vi "引用測試2.vi"() -> ()   [LabVIEW 2015]
uses:
  <vilib>/vision/Measure.llb/Edge Options.ctl
  <vilib>/vision/Measure.llb/Edge Polarity.ctl
  <vilib>/userdefined/High Color/IMAQdx.ctl
  <vilib>/vision/driver/NI_Vision_Acquisition_Software.lvlib
  <vilib>/vision/NI_Vision_Development_Module.lvlib
panel:
  in  "Boolean":bool
  out "Line Data":T1
  in  "取像":bool
  in  "Edge Options":T2={"Edge Polarity"=0, "Kernel Size"=3, "Width"=3, "Minimum Edge Strength"=10.0, "Interpolation Type"=enum."Bilinear Fixed", "Data Processing Method"=enum."Average"} {"Edge Polarity" items=["All Edges", "Rising Edges", "Falling Edges"]; "Minimum Edge Strength" format="%.2f"; "Width" step=2; "Kernel Size" step=2}
  out "error out":errorcluster
  out "Ellipse":T4 {"Minor Axis"."Point 2"."Y" format="%.2f"; "Minor Axis"."Point 2"."X" format="%.2f"; "Minor Axis"."Point 1"."Y" format="%.2f"; "Minor Axis"."Point 1"."X" format="%.2f"; "Major Axis"."Point 2"."Y" format="%.2f"; "Major Axis"."Point 2"."X" format="%.2f"; "Major Axis"."Point 1"."Y" format="%.2f"; "Major Axis"."Point 1"."X" format="%.2f"; "Center"."Y" format="%.2f"; "Center"."X" format="%.2f"}
  in  "圓":enum16{"Inner to Outer", "Outer to Inner"}(ring)
  out "Gradient Information":dbl[][](graph)
  in  "邊":T5(ring)
  in  "Process":T6(ring)
  in  "Gap":i32=10 min=1 max=300
  in  "stop":bool
  out "Image":T7(plugin-control)
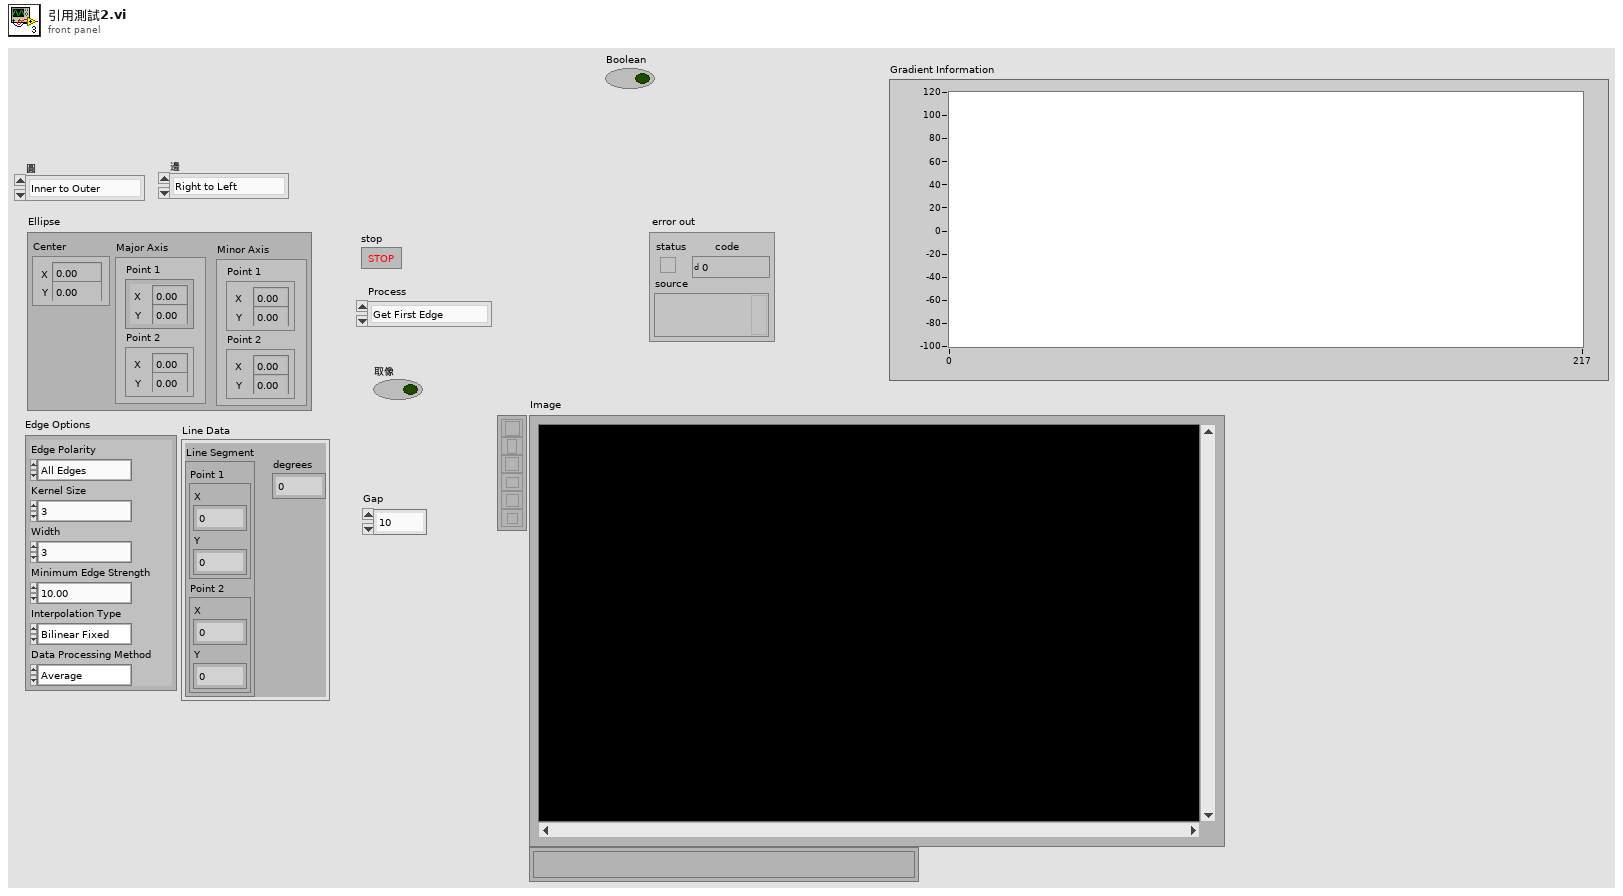
[diagram p1: front panel]
types:
  T1 = cluster{"Line Segment":cluster{"Point 1":cluster{"X":sgl, "Y":sgl}, "Point 2":cluster{"X":sgl, "Y":sgl}}, "degrees":sgl}
  T2 = typedef "Edge Options.ctl" = cluster{"Edge Polarity":T3, "Kernel Size":u32, "Width":u32, "Minimum Edge Strength":sgl, "Interpolation Type":enum32{"Zero Order", "Bilinear", "Quadratic", "Cubic", "Bilinear Fixed"}, "Data Processing Method":enum32{"Average", "Median"}}
  T3 = typedef "Edge Polarity.ctl" = u32
  T4 = cluster{"Center":cluster{"X":sgl, "Y":sgl}, "Major Axis":cluster{"Point 1":cluster{"X":sgl, "Y":sgl}, "Point 2":cluster{"X":sgl, "Y":sgl}}, "Minor Axis":cluster{"Point 1":cluster{"X":sgl, "Y":sgl}, "Point 2":cluster{"X":sgl, "Y":sgl}}}
  T5 = enum16{"Right to Left", "Left  to Right", "Up to Down", "Down to Up"}
  T6 = enum16{"Get First Edge", "Get First + Last Edge", "Get All Edges", "Get Best Edge"}
  T7 = typedef "IMAQ Image.ctl" = refnum<image>
  T8 = typedef "IMAQdx.ctl" = refnum<k21>
  T9 = typedef "Image Type" = u32
  T10 = cluster{"Global Rectangle":i32[], "Contours":cluster{"Contour Type":u32, "ROI Type":u32, "Points":i32[]}[]}
  T11 = cluster{"Contour Type":u32, "ROI Type":u32, "Points":i32[]}[]
  T12 = cluster{"Contour Type":u32, "ROI Type":u32, "Points":i32[]}
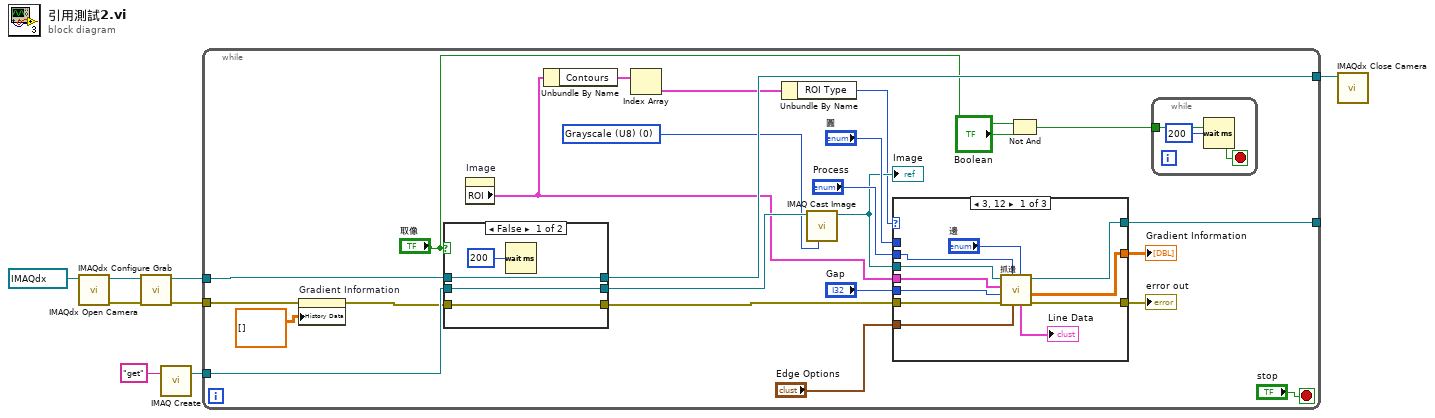
[diagram p0: block diagram]
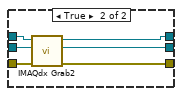
[diagram p2: hidden frame]
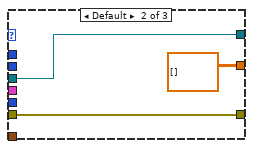
[diagram p3: hidden frame]
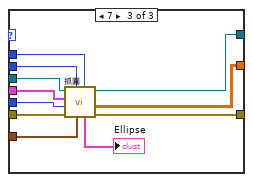
[diagram p4: hidden frame]
diagram:
  n1 = call <vilib>:"IMAQdx Open Camera.vi"("Session In"=T8 "cam1") -> ("error out"=w1:errorcluster, "Session Out"=w2:T8)  [unwired: 9 in]
  n2 = call <vilib>:"IMAQdx Configure Grab.vi"("error in"=w1, "Session In"=w2) -> ("error out"=w5:errorcluster, "Session Out"=w7:T8)  [unwired: 8 in]
  n3 = call "IMAQ Create"("Image Name"="get") -> ("New Image"=w6:T7)  [unwired: 4 in, 1 out]
  n4 = while {
    tunnel: w7 -> [w33]
    tunnel: w6 -> [w32]
    tunnel: w5 -> [w25]
    tunnel: [w30] -> w4
    tunnel: [w19] -> _
    stop <- "stop" stop-if-true
    w28 = T9 0 items=["Grayscale (U8)", "Grayscale (I16)", "Grayscale (SGL)", "Complex (CSG)", "RGB (U32)", "HSL (U32)", "RGB (U64)", "Grayscale (U16)"] ("Image Type")
    n5 = property on="Gradient Information" class="WFChart (strict)"(error in=w25, "History Data"=dbl[][] []) -> (error out=w26:errorcluster)  [unwired: 1 in, 1 out]
    n6 = case shown="False" "取像" {
      tunnel: w33 -> [w39 w45]
      tunnel: w32 -> [w38 w44]
      tunnel: [w39 w43] -> w30
      tunnel: [w38 w42] -> w29
      tunnel: w26 -> [w37 w41]
      tunnel: [w37 w40] -> w23
      frame False {
        n7 = Wait (ms)(milliseconds to wait=u32 200) -> ()  [unwired: 1 out]
      }
      frame True {
        n8 = call <vilib>:"IMAQdx Grab2.vi"("error in"=w41, "Image In"=w44, "Session In"=w45) -> ("error out"=w40:errorcluster, "Image Out"=w42:T7, "Session Out"=w43:T8)  [unwired: 5 in, 1 out]
      }
    }
    n9 = property on="Image" class="ImageControl"() -> ("ROI"=w17:T10)  [unwired: 2 in, 2 out]
    n10 = Unbundle By Name(w17) -> ("Contours"=w16:T11)
    n11 = Index Array(array=w16) -> (element=w15:T12)  [unwired: 1 in]
    n12 = Unbundle By Name(w15) -> ("ROI Type"=w14:u32)
    n13 = call "IMAQ Cast Image"("Image Type"=w28, "Image Src"=w29) -> ("Image Dst Out"=w20:T7)  [unwired: 8 in, 1 out]
    "Image" <- w20
    n14 = case shown="3, 12" w14 {
      tunnel: w17 -> [w52 _ w70]
      tunnel: "Gap" -> [w51 _ w69]
      tunnel: w23 -> [w50 w57 w68]
      tunnel: "圓" -> [_ _ w67]
      tunnel: "Process" -> [w53 _ w66]
      tunnel: [w48 dbl[][] [] ("Gradient Information") w65] -> w12
      tunnel: w20 -> [w56 w59 w64]
      tunnel: [w55 w59 w62] -> w19
      tunnel: [w49 w57 w61] -> w18
      tunnel: "Edge Options" -> [w47 _ w60]
      frame 3, 12 {
        n15 = call "抓邊.vi"("Direction"="邊", "Edge Options"=w47, "Process"=w53, "error In"=w50, "Gap"=w51, "ROI"=w52, "Image In"=w56) -> ("error out"=w49:errorcluster, "Gradient Information"=w48:dbl[][], "Image"=w55:T7, "Line Data"=→"Line Data":T1)  [unwired: 1 out]
      }
      frame Default {
      }
      frame 7 {
        n16 = call "抓圓.vi"("Direction"=w67, "Edge Options"=w60, "Process"=w66, "error In"=w68, "Gap"=w69, "ROI"=w70, "Image In"=w64) -> ("error out"=w61:errorcluster, "Gradient Information"=w65:dbl[][], "Image"=w62:T7, "Ellipse"=→"Ellipse":T4)  [unwired: 1 out]
      }
    }
    "error out" <- w18
    "Gradient Information" <- w12
    n17 = Not And(1:"Boolean", 2:"取像") -> (0:w9:bool)
    n18 = while {
      tunnel: w9 -> [w35]
      stop <- w35 stop-if-true
      n19 = Wait (ms)(milliseconds to wait=u32 200) -> ()  [unwired: 1 out]
    }
  }
  n20 = call <vilib>:"IMAQdx Close Camera.vi"("Session In"=w4) -> ()  [unwired: 10 in, 1 out]
